vi "Init_Programmer.vi"(8 "error in (no error)":errorcluster, 11 "IN":T1={"step name 1"="", "updata 2"="1000", "limitdata 3"="", "load vi name 4"="", "parameter 5"=""}) -> (0 "error out":errorcluster, 3 "Cluster":T2)   [LabVIEW 2013]
uses:
  Sub vi/Global constant.vi
panel:
  out "type string":i16[](array[numeric])
  out "data string":string
  out "GetMainHardwareID":variant
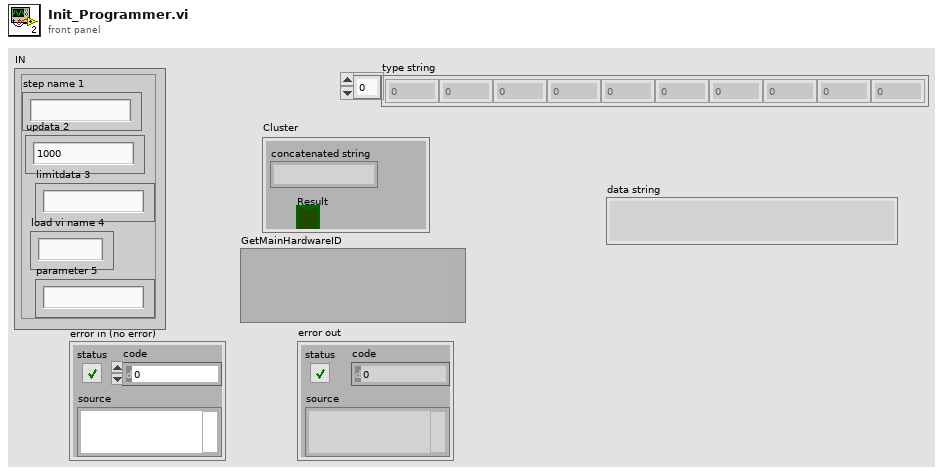
[diagram p1: front panel]
types:
  T1 = cluster{"step name 1":string, "updata 2":string, "limitdata 3":string, "load vi name 4":string, "parameter 5":string}
  T2 = cluster{"concatenated string":string, "Result":bool}
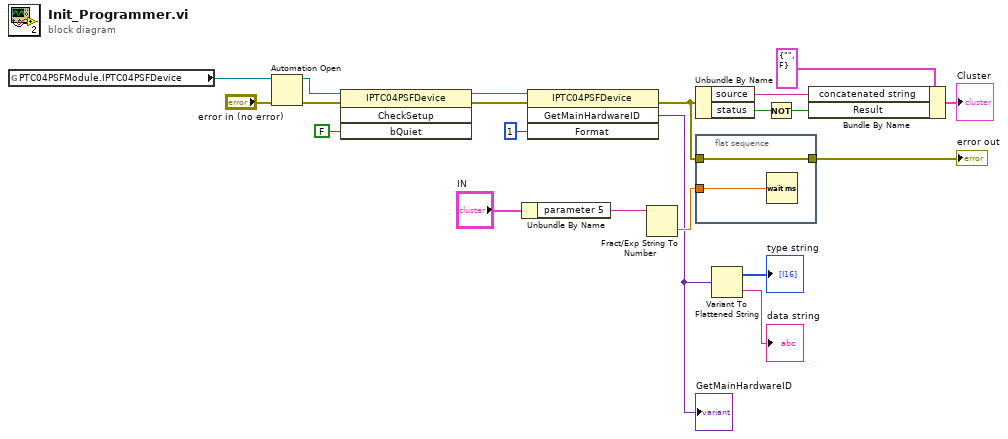
[diagram p0: block diagram]
diagram:
  n1 = global read "Global constant.vi" "PTC04PSFModule.IPTC04PSFDevice"() -> (w16:refnum<k7>)
  n2 = Automation Open(error in (no error)="error in (no error)", Automation Refnum=w16) -> (Automation Refnum=w14:refnum<k7>, error out=w13:errorcluster)  [unwired: 2 in]
  n3 = invoke class="IPTC04PSFDevice" method="CheckSetup"(reference=w14, error in=w13, "bQuiet"=FALSE) -> (reference out=w7:refnum<k7>, error out=w6:errorcluster)  [unwired: 1 in, 2 out]
  n4 = Unbundle By Name("IN") -> ("parameter 5"=w17:string)
  n5 = invoke class="IPTC04PSFDevice" method="GetMainHardwareID"(reference=w7, error in=w6, "Format"=1) -> (error out=w4:errorcluster, "GetMainHardwareID"=w3:variant)  [unwired: 1 in, 2 out]
  "GetMainHardwareID" <- w3
  n6 = Fract/Exp String To Number(string=w17) -> (number=w18:dbl)  [unwired: 3 in, 1 out]
  n7 = Unbundle By Name(w4) -> ("source"=w9:string, "status"=w11:bool)
  n8 = flat-sequence {
    tunnel: w18 -> [w23]
    tunnel: w4 -> [w22]
    tunnel: [w22] -> w8
    frame #0 {
      n9 = Wait (ms)(milliseconds to wait=w23) -> ()  [unwired: 1 out]
    }
  }
  n10 = Variant To Flattened String(Variant=w3) -> (data string=→"data string":string, 1:→"type string":i16[])
  n11 = Not(x=w11) -> (.not. x?=w10:bool)
  n12 = Bundle By Name(cluster=T2 {"concatenated string"="", "Result"=FALSE} ("Cluster"), "concatenated string"=w9, "Result"=w10) -> (→"Cluster":T2)
  "error out" <- w8
